vi "ucno_formula string function.vi"(3 "output control":T1, 4 "data":variant, 5 "X":dbl[](array[numeric])) -> (0 "error out":errorcluster, 1 "gradient":dbl[](array[numeric]), 2 "f(X)":dbl)   [LabVIEW 2020, in "NI_Gmath.lvlib"]
uses:
  <vilib>/gmath/NI_Gmath.lvlib
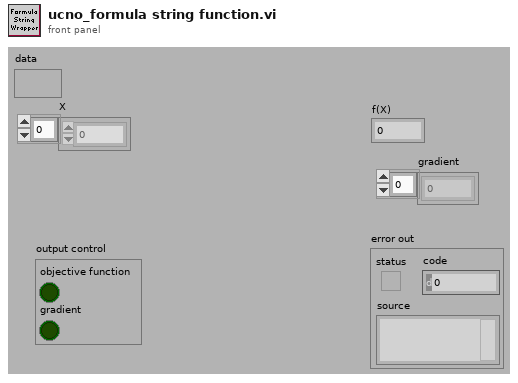
[diagram p1: front panel]
types:
  T1 = cluster{"objective function":bool, "gradient":bool}
  T2 = cluster{"objective function":string, "X":string[]}
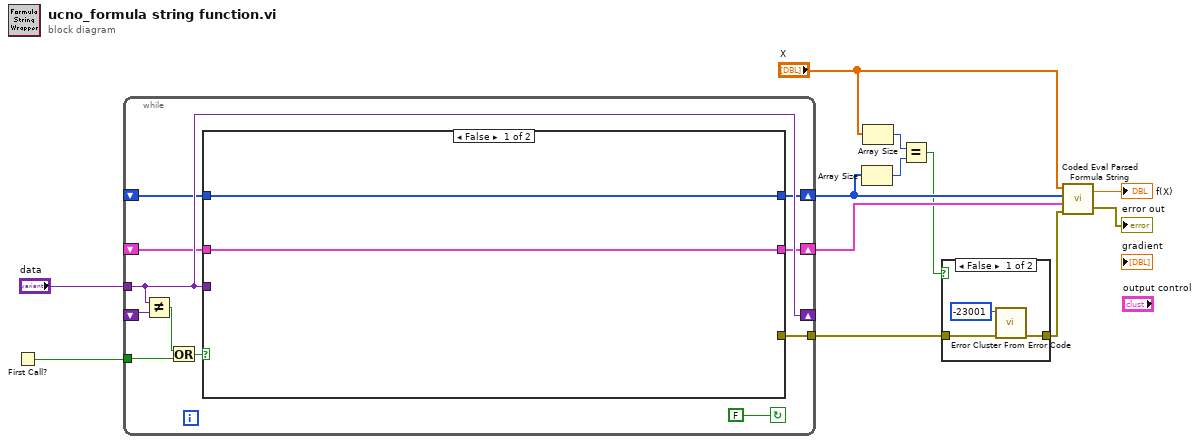
[diagram p0: block diagram]
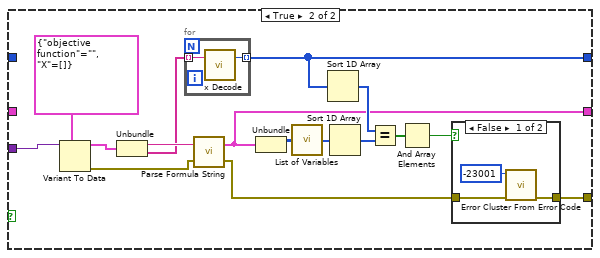
[diagram p3: hidden frame]
diagram:
  n1 = First Call?() -> (First Call?: T/F=w12:bool)
  n2 = while {
    shift-right: [w19] -> w5
    shift-left: _ -> [w21]
    shift-right: [w22] -> w10
    shift-left: _ -> [w20]
    tunnel: w12 -> [w14]
    tunnel: "data" -> [w23]
    tunnel: [w17] -> w3
    shift-right: [w23] -> _
    shift-left: _ -> [w16]
    stop <- FALSE continue-if-true
    n3 = Not Equal?(x=w23, y=w16) -> (x != y?=w15:bool)
    n4 = Or(x=w15, y=w14) -> (x .or. y?=w13:bool)
    n5 = case shown="False" w13 {
      tunnel: w23 -> [_ w34]
      tunnel: [w24 w33] -> w22
      tunnel: w21 -> [w25 _]
      tunnel: w20 -> [w24 _]
      tunnel: [w25 w32] -> w19
      tunnel: [_ w27] -> w17
      frame False {
      }
      frame True {
        n6 = Variant To Data(type=T2 {"objective function"="", "X"=[]}, Variant=w34) -> (data=w37:T2, error out=w30:errorcluster)  [unwired: 1 in]
        n7 = Unbundle(w37) -> ("objective function"=w36:string, "X"=w31:string[])
        n8 = for {
          tunnel: w31 -> [w47] mode=indexing
          tunnel: [w46] -> w33 mode=indexing
          n9 = call <vilib>:"x Decode.vi"("x string"=w47) -> ("number"=w46:i32)  [unwired: 1 in, 1 out]
        }
        n10 = call <vilib>:"Parse Formula String.vi"("error in (no error)"=w30, "formula"=w36) -> ("error out"=w26:errorcluster, "Parsed Formula"=w32:cluster{"Table":i32[][], "Y Values":dbl[]})
        n11 = Unbundle(w32) -> ("Table"=w35:i32[][])  [unwired: 1 out]
        n12 = call <vilib>:"List of Variables.vi"("Table"=w35) -> ("List of variables"=w40:i32[])
        n13 = Sort 1D Array(array=w33) -> (sorted array=w41:i32[])
        n14 = Sort 1D Array(array=w40) -> (sorted array=w29:i32[])
        n15 = Equal?(x=w41, y=w29) -> (x = y?=w39:bool[])
        n16 = And Array Elements(Boolean array=w39) -> (logical AND=w28:bool)
        n17 = case shown="False" w28 {
          tunnel: w26 -> [w43 w45]
          tunnel: [w42 w45] -> w27
          frame False {
            n18 = call <vilib>:"Error Cluster From Error Code.vi"("error in (no error)"=w43, "error code (0)"=-23001) -> ("error out"=w42:errorcluster)  [unwired: 7 in]
          }
          frame True {
          }
        }
      }
    }
  }
  n19 = Array Size(array=w10) -> (size(s)=w7:i32)
  n20 = Array Size(array="X") -> (size(s)=w8:i32)
  n21 = Equal?(x=w8, y=w7) -> (x = y?=w4:bool)
  n22 = case shown="False" w4 {
    tunnel: w3 -> [w49 w51]
    tunnel: [w48 w51] -> w2
    frame False {
      n23 = call <vilib>:"Error Cluster From Error Code.vi"("error in (no error)"=w49, "error code (0)"=-23001) -> ("error out"=w48:errorcluster)  [unwired: 7 in]
    }
    frame True {
    }
  }
  n24 = call <vilib>:"Coded Eval Parsed Formula String.vi"("error in (no error)"=w2, "Parsed Formula"=w5, "Variables"=w10, "X Values"="X") -> ("error out"=→"error out":errorcluster, "y value"=→"f(X)":dbl)
